vi "compareArrayDataCoil.vi"(9 "B":variant, 10 "A":variant) -> (1 "Value":bool, 2 "BitChange":i32, 3 "Enum":T1(ring))   [LabVIEW 2014]
doc: "So sanh 2 Array Data\n- Type data : Boolean.\nReturn:\n- Index array change.\n- value of index array."
panel:
  in  "DataCoil":bool[](array[boolean])
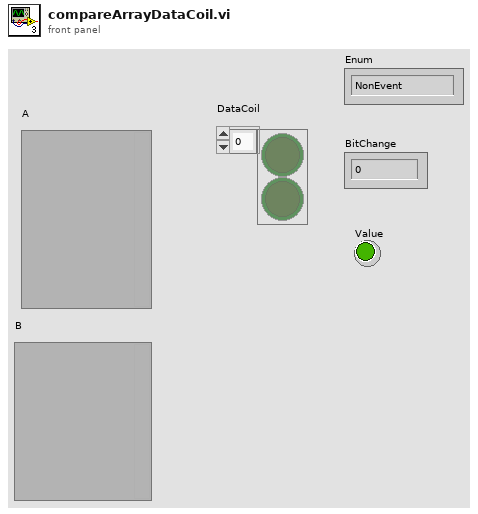
[diagram p1: front panel]
types:
  T1 = enum16{"NonEvent", "EMG", "X+", "X-", "Y+", "Y-", "Z+", "Z-", "Mode", "GoHome", "StartAuto", "SaveEprom", "SetAccel", "SetFeedRate", "SetStepSize", "SetStartAccel", "ResetError", "AddG0", "AddG1", "AddSoleNoid", "AddPWM", "AddFan", "WaitInput", "AddSpin", "ControlSpin"}
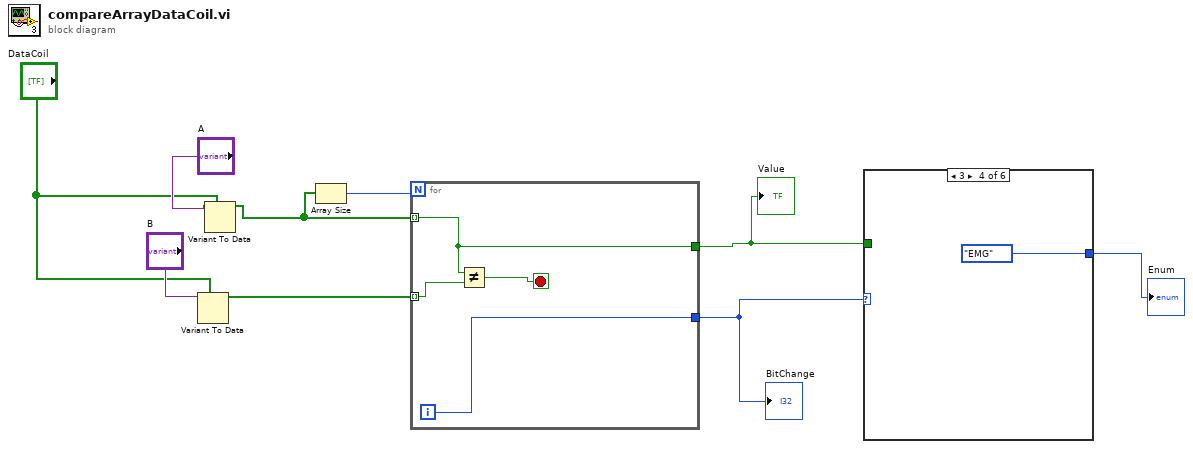
[diagram p0: block diagram]
diagram:
  n1 = Variant To Data(type="DataCoil", Variant="B") -> (data=w7:bool[])  [unwired: 1 in, 1 out]
  n2 = Variant To Data(type="DataCoil", Variant="A") -> (data=w6:bool[])  [unwired: 1 in, 1 out]
  n3 = Array Size(array=w6) -> (size(s)=w5:i32)
  n4 = for {
    N: w5 -> [_]
    tunnel: w6 -> [w10] mode=indexing
    tunnel: w7 -> [w13] mode=indexing
    tunnel: [w11] -> w3
    tunnel: [w10] -> w2
    i -> [w11]
    stop <- w12 stop-if-true
    n5 = Not Equal?(x=w10, y=w13) -> (x != y?=w12:bool)
  }
  "BitChange" <- w3
  "Value" <- w2
  n6 = case shown="3" w3 {
    tunnel: w2 -> [_ _ _ _ _ _]
    tunnel: [_ _ _ T1."EMG" ("Enum") _ _] -> w1
    frame 0, Default {
    }
    frame 1 {
    }
    frame 2 {
    }
    frame 3 {
    }
    frame 4 {
    }
    frame 5 {
    }
  }
  "Enum" <- w1
